vi "Do.vi"(8 "error in (no error)":errorcluster, 10 "Actor in":refnum<class "Actor.lvclass">, 11 "Measure Msg":refnum<class "Measure Msg.lvclass">) -> (0 "error out":errorcluster, 2 "Actor out":refnum<class "Actor.lvclass">)   [LabVIEW 2021, in "Measure Msg.lvclass"]
doc: "This VI delivers the message to the actor by calling the appropriate method(s) on the actor."
uses:
  Measure Msg.lvclass
  Measure Msg.lvclass/Measure Msg.ctl
  2d5e62c2-8a4b-47e0-a91d-c47d7f903c68.vi
  Continuous Recorder/Continuous Recorder.lvclass
  <vilib>/ActorFramework/Actor/Actor.lvclass
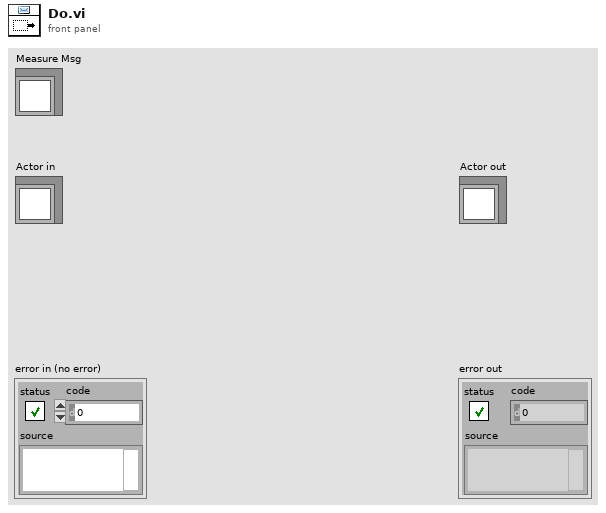
[diagram p1: front panel]
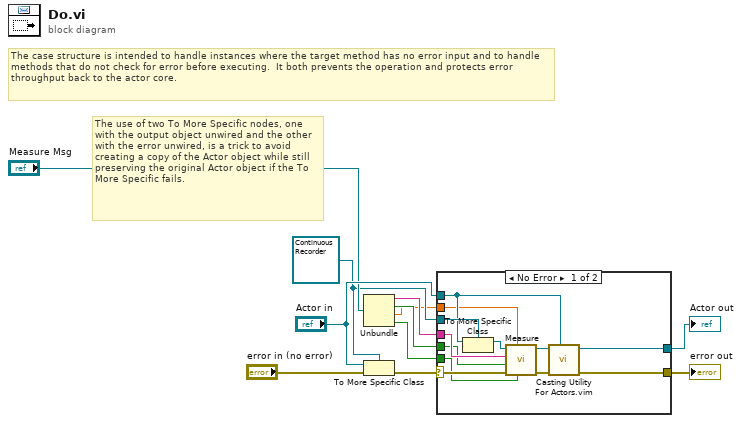
[diagram p0: block diagram]
diagram:
  w6 = refnum<class "Continuous Recorder.lvclass"> refnum ("Actor in")
  # "The use of two To More Specific nodes, one with the output object unwired and the other with the error unwired, is a trick to avoid creating a copy of the Actor object while still preserving the original Actor object if the To More Specific fails."
  # "The case structure is intended to handle instances where the target method has no error input and to handle methods that do not check for error before executing.  It both prevents the operation and protects error throughput back to the actor core."
  n1 = Unbundle("Measure Msg") -> (w4:string, w3:bool, w2:dbl, w1:bool)
  n2 = To More Specific Class(target class=w6, reference="Actor in", error in="error in (no error)") -> (error out=w5:errorcluster)  [unwired: 1 out]
  n3 = case shown="No Error" w5 {
    selector: w5 -> [w23 w25]
    tunnel: [w17 w25] -> w11
    tunnel: [w18 w24] -> w10
    tunnel: "Actor in" -> [w20 w24]
    tunnel: w6 -> [w21 _]
    tunnel: w4 -> [w15 _]
    tunnel: w3 -> [w14 _]
    tunnel: w2 -> [w13 _]
    tunnel: w1 -> [w12 _]
    frame No Error {
      n4 = To More Specific Class(target class=w21, reference=w20) -> (specific class reference=w22:refnum<class "Continuous Recorder.lvclass">)  [unwired: 1 in, 1 out]
      n5 = call-dynamic "Measure.vi"("Init work"=w12, "Update period"=w13, "error in (no error)"=w23, "Last request"=w14, "Requester"=w15, "Continuous Recorder in"=w22) -> ("error out"=w16:errorcluster, "Continuous Recorder out"=w19:refnum<class "Continuous Recorder.lvclass">)  [unwired: 4 in]
      n6 = call "Casting Utility For Actors.vim"("type"=w20, "error in (no error)"=w16, "Actor in"=w19) -> ("error out"=w17:errorcluster, "Actor out"=w18:refnum<class "Actor.lvclass">)  [unwired: 7 in]
    }
    frame Error {
      # "If type check fails, pass the original object out again."
    }
  }
  "error out" <- w11
  "Actor out" <- w10
